vi "Configure Channel Basic.vi"(0 "VISA resource name":refnum<visa-resource-name>, 1 "Enable Channel (F: Disable)":bool, 2 "Probe":i32(ring)=12 items=["0.001", "0.002", "0.005", "0.01", "0.02", "0.05", "0.1", "0.2", "0.5", "1", "2", "5", "10", "20", "50", "100", "200", "500", "1000"], 3 "Enable Inverted Display (F: Disable)":bool, 5 "Channel (1: Channel 1)":i32(ring)=1 items=["Channel 1"=1, "Channel 2"=2, "Channel 3"=3, "Channel 4"=4], 7 "Bandwidth Limit":i32(ring)=1 items=["20M", "Off"], 9 "Coupling Mode (1: DC)":i32(ring)=1 items=["AC", "DC", "GND"], 11 "error in (no error)":errorcluster, 12 "Unit (0: Voltage)":i32(ring) items=["Voltage", "Ampere"]) -> (4 "VISA resource name out":refnum<visa-resource-name>, 15 "error out":errorcluster)   [LabVIEW 2015]
doc: "Configures the basic setting for channel."
uses:
  ZhiYuan ZDS Series for TCP.lvlib
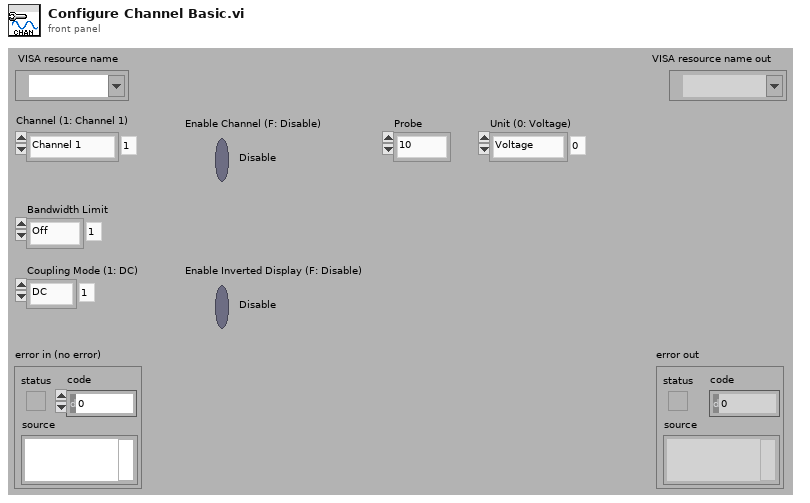
[diagram p1: front panel]
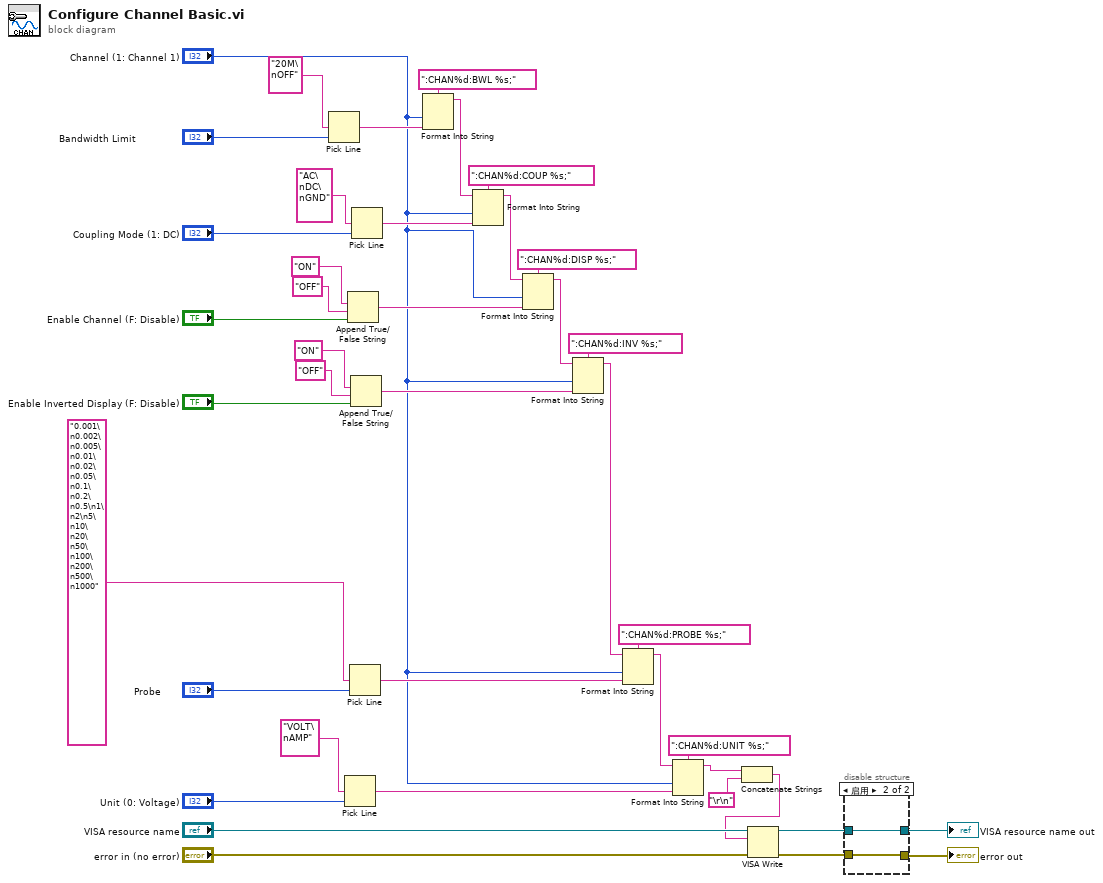
[diagram p0: block diagram]
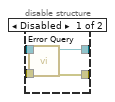
[diagram p2: hidden frame]
diagram:
  n1 = Pick Line(multi-line string="20M\nOFF", line index="Bandwidth Limit") -> (output string=w38:string)  [unwired: 1 in]
  n2 = Pick Line(multi-line string="VOLT\nAMP", line index="Unit (0: Voltage)") -> (output string=w13:string)  [unwired: 1 in]
  n3 = Append True/False String(1:"Enable Channel (F: Disable)", 2:"OFF", 3:"ON") -> (0:w27:string)  [unwired: 1 in]
  n4 = Pick Line(multi-line string="0.001\n0.002\n0.005\n0.01\n0.02\n0.05\n0.1\n0.2\n0.5\n1\n2\n5\n10\n20\n50\n100\n200\n500\n1000", line index="Probe") -> (output string=w17:string)  [unwired: 1 in]
  n5 = Append True/False String(1:"Enable Inverted Display (F: Disable)", 2:"OFF", 3:"ON") -> (0:w21:string)  [unwired: 1 in]
  n6 = Pick Line(multi-line string="AC\nDC\nGND", line index="Coupling Mode (1: DC)") -> (output string=w33:string)  [unwired: 1 in]
  n7 = Format Into String(format string=":CHAN%d:BWL %s;", "Channel (1: Channel 1)", w38) -> (resulting string=w35:string)  [unwired: 2 in, 1 out]
  n8 = Format Into String(format string=":CHAN%d:COUP %s;", initial string=w35, "Channel (1: Channel 1)", w33) -> (resulting string=w29:string)  [unwired: 1 in, 1 out]
  n9 = Format Into String(format string=":CHAN%d:DISP %s;", initial string=w29, "Channel (1: Channel 1)", w27) -> (resulting string=w23:string)  [unwired: 1 in, 1 out]
  n10 = Format Into String(format string=":CHAN%d:INV %s;", initial string=w23, "Channel (1: Channel 1)", w21) -> (resulting string=w5:string)  [unwired: 1 in, 1 out]
  n11 = Format Into String(format string=":CHAN%d:PROBE %s;", initial string=w5, "Channel (1: Channel 1)", w17) -> (resulting string=w4:string)  [unwired: 1 in, 1 out]
  n12 = Format Into String(format string=":CHAN%d:UNIT %s;", initial string=w4, "Channel (1: Channel 1)", w13) -> (resulting string=w3:string)  [unwired: 1 in, 1 out]
  n13 = Concatenate Strings(w3, "\r\n") -> (w1:string)
  n14 = VISA Write(VISA resource name="VISA resource name", write buffer=w1, error in (no error)="error in (no error)") -> (VISA resource name out=w10:refnum<visa-resource-name>, error out=w9:errorcluster)  [unwired: 1 out]
  n15 = disable-structure shown="启用" {
    disable-tunnel: w10 -> [w45 w47]
    disable-tunnel: w9 -> [w44 w46]
    disable-tunnel: [w43 w47] -> w8
    disable-tunnel: [w42 w46] -> w7
    frame Disabled {
      n16 = call "Error Query.vi"("error in (no error)"=w44, "VISA resource name"=w45) -> ("error out"=w42:errorcluster, "VISA resource name out"=w43:refnum<visa-resource-name>)  [unwired: 6 in, 2 out]
    }
    frame Enabled {
    }
  }
  "VISA resource name out" <- w8
  "error out" <- w7
